vi "CLC_Single_Channel_CMD.vi"(7 "Channel params":T1={"Mode"=1, "Polarity"=1, "CH_ON/OFF"=1, "Channel"=0, "Gain"=0, "Phase"=0} {"CH_ON/OFF" items=["ON", "OFF"]; "Polarity" items=["H", "V"]; "Mode" items=["Tx"=1, "Rx"=2]}, 8 "error in":errorcluster, 11 "TCPIPin":T2={"address"="192.168.100.111", "remote port or service name"=5025, "timeout ms (60000)"=10000}) -> (0 "error out":errorcluster, 1 "OK?":bool, 3 "TCPIPout":T2={"address"="192.168.100.111", "remote port or service name"=5025, "timeout ms (60000)"=10000})   [LabVIEW 2023]
panel:
  out "data out":string
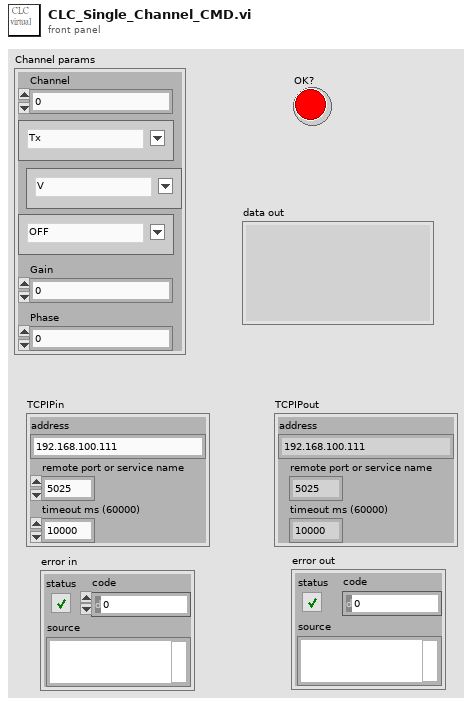
[diagram p1: front panel]
types:
  T1 = cluster{"Mode":u16, "Polarity":u16, "CH_ON/OFF":u16, "Channel":i32, "Gain":i32, "Phase":i32}
  T2 = cluster{"address":string, "remote port or service name":u16, "timeout ms (60000)":i32}
  T3 = enum16{"Standard", "Buffered", "CRLF", "Immediate"}
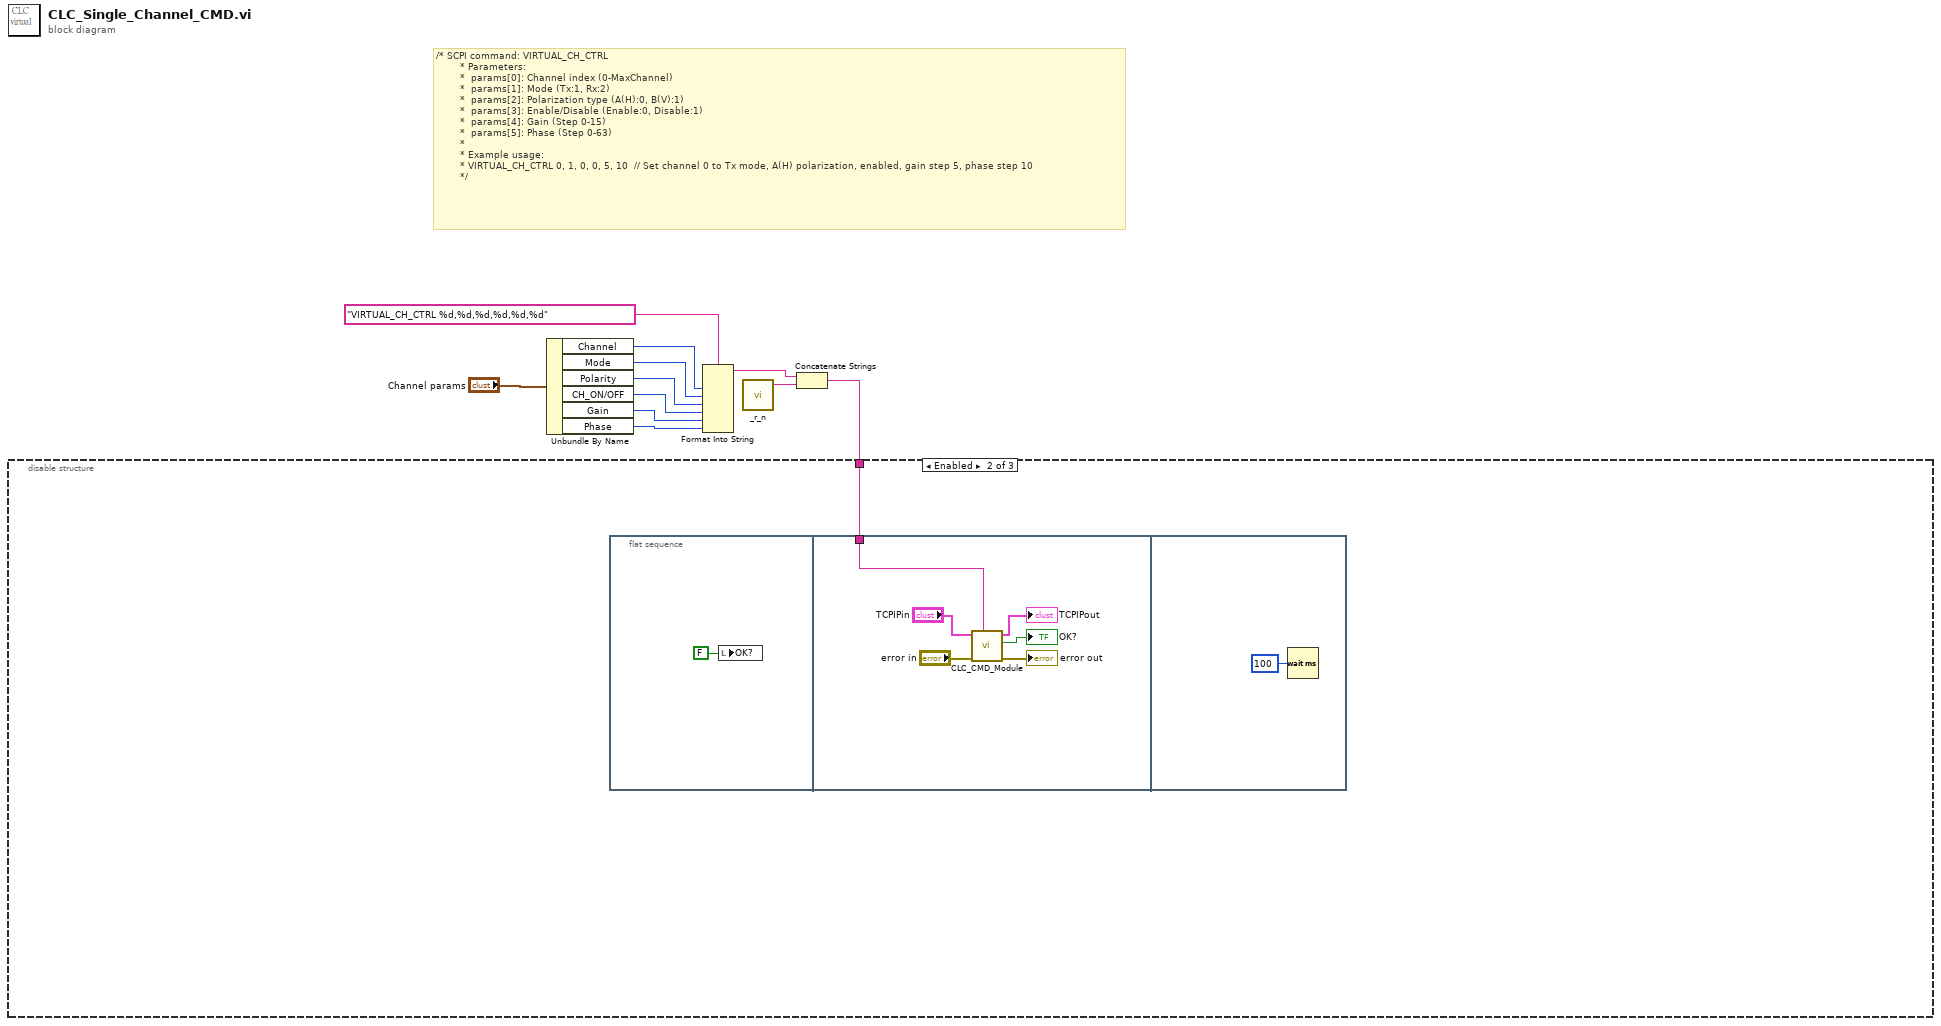
[diagram p0: block diagram]
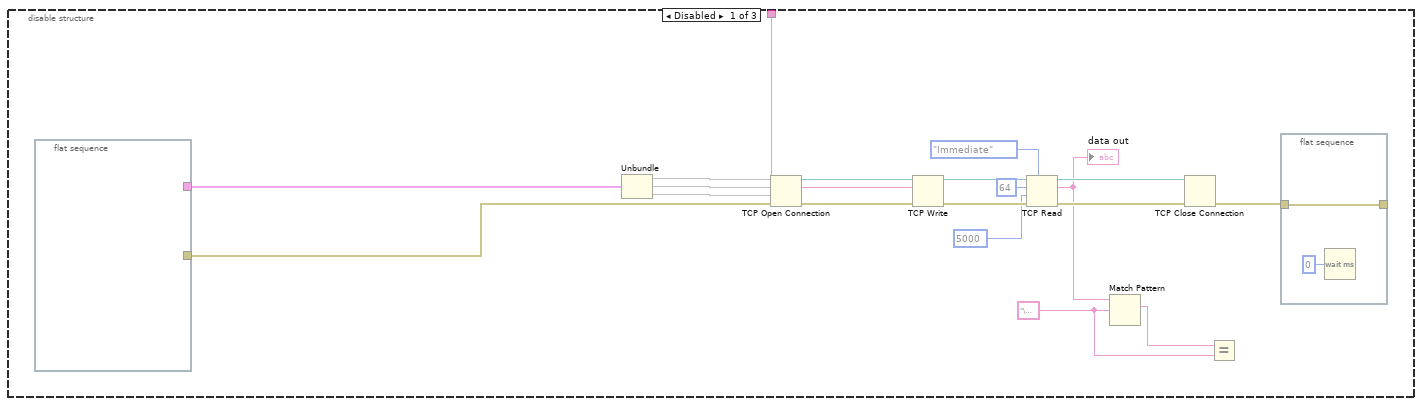
[diagram p2: hidden frame]
diagram:
  # "/* SCPI command: VIRTUAL_CH_CTRL\n        * Parameters:\n        *  params[0]: Channel index (0-MaxChannel)\n        *  params[1]: Mode (Tx:1, Rx:2)\n        *  params[2]: Polarization type (A(H):0, B(V):1)\n        *  params[3]: Enable/Disable (Enable:0, Disable:1)\n        *  params[4]: Gain (Step 0-15)\n        *  params[5]: Phase (Step 0-63)\n        * \n        * Example usage:\n        * VIRTUAL_CH_CTRL 0, 1, 0, 0, 5, 10  // Set channel 0 to Tx mode, A(H) polarization, enabled, gain step 5, phase step 10\n        */"
  n1 = Unbundle By Name("Channel params") -> ("Channel"=w6:i32, "Mode"=w5:u16, "Polarity"=w4:u16, "CH_ON/OFF"=w3:u16, "Gain"=w2:i32, "Phase"=w1:i32)
  n2 = Format Into String(format string="VIRTUAL_CH_CTRL %d,%d,%d,%d,%d,%d" ("data in"), w6, w5, w4, w3, w2, w1) -> (resulting string=w9:string)  [unwired: 2 in, 1 out]
  n3 = call "_r_n.vi"() -> ("command"=w8:string)  [unwired: 5 in]
  n4 = Concatenate Strings(w9, w8) -> (w11:string)
  n5 = disable-structure shown="Enabled" {
    disable-tunnel: w11 -> [w26 w33 _]
    frame Disabled {
      w13 = "\u0000" ("string")
      n6 = flat-sequence {
        tunnel: [_] -> w30
        tunnel: [_] -> w29
        frame #0 {
        }
      }
      n7 = Unbundle(w30) -> ("address"=w25, "remote port or service name"=w24, "timeout ms (60000)"=w23)
      n8 = TCP Open Connection(address=w25, remote port or service name=w24, timeout ms (60000)=w23, error in (no error)=w29) -> (connection ID=w28:refnum<k5>, error out=w27:errorcluster)  [unwired: 1 in]
      n9 = TCP Write(connection ID=w28, data in=w26, error in (no error)=w27) -> (connection ID out=w21:refnum<k5>, error out=w22:errorcluster)  [unwired: 1 in, 1 out]
      n10 = TCP Read(connection ID=w21, bytes to read=64, error in (no error)=w22, 7:T3."Immediate" ("mode (standard)"), 9:5000 ("timeout ms (25000)")) -> (connection ID out=w20:refnum<k5>, data out=w15:string, error out=w19:errorcluster)
      "data out" <- w15
      n11 = Match Pattern(string=w15, regular expression=w13) -> (match substring=w14:string)  [unwired: 1 in, 3 out]
      n12 = TCP Close Connection(connection ID=w20, error in (no error)=w19) -> (error out=w12:errorcluster)  [unwired: 1 in, 1 out]
      n13 = Equal?(x=w14, y=w13) -> ()  [unwired: 1 out]
      n14 = flat-sequence {
        tunnel: w12 -> [w32]
        tunnel: [w32] -> _
        frame #0 {
          n15 = Wait (ms)(milliseconds to wait=u32 0) -> ()  [unwired: 1 out]
        }
      }
    }
    frame Enabled {
      n16 = flat-sequence {
        tunnel: w33 -> [w38]
        frame #0 {
          n17 = local write "OK?"(FALSE ("OK?")) -> ()
        }
        frame #1 {
          n18 = call "CLC_CMD_Module.vi"("CMD in"=w38, "error in"="error in", "TCPIPin"="TCPIPin") -> ("error out"=→"error out":errorcluster, "OK?"=→"OK?":bool, "TCPIPout"=→"TCPIPout":T2)  [unwired: 5 in, 1 out]
        }
        frame #2 {
          n19 = Wait (ms)(milliseconds to wait=u32 100) -> ()  [unwired: 1 out]
        }
      }
    }
    frame Disabled {
    }
  }
